vi "Initialize.vi"(8 "error in (no error)":errorcluster, 11 "SingleB in":refnum<class "SingleB.lvclass">) -> (0 "error out":errorcluster, 3 "SingleB out":refnum<class "SingleB.lvclass">)   [LabVIEW 2020, in "SingleB.lvclass"]
uses:
  SingleB.lvclass
  D:/03 GitHub/LabVIEW-Singleton/Singleton/Singleton.lvclass
  Singleton/Singleton.lvclass
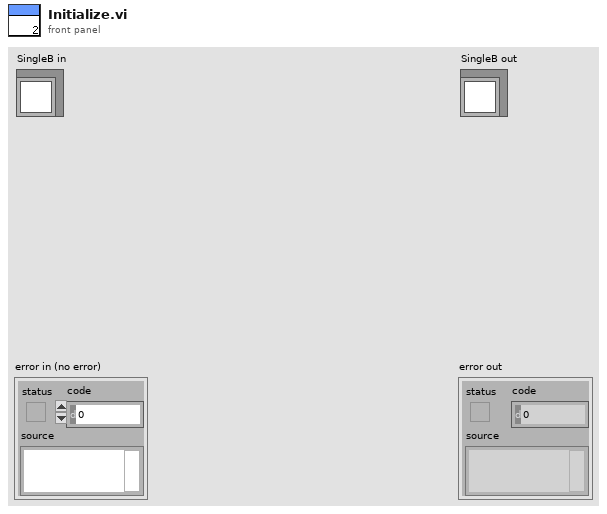
[diagram p1: front panel]
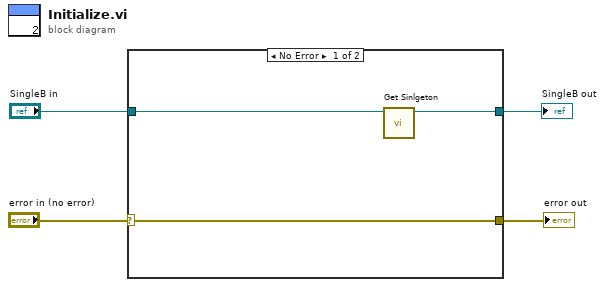
[diagram p0: block diagram]
diagram:
  n1 = case shown="No Error" "error in (no error)" {
    selector: "error in (no error)" -> [w7 w9]
    tunnel: [w7 w9] -> w2
    tunnel: "SingleB in" -> [w6 w8]
    tunnel: [w5 w8] -> w3
    frame No Error {
      n2 = call "Get Sinlgeton.vi"("Singleton in"=w6) -> ("Singleton out"=w5:refnum<class "SingleB.lvclass">)  [unwired: 10 in]
    }
    frame Error {
    }
  }
  "error out" <- w2
  "SingleB out" <- w3
